vi "ex5_for loop.vi"() -> ()   [LabVIEW 2018]
panel:
  out "Numeric 2":dbl
  out "Array":dbl[](array[numeric])
  out "Numeric":dbl
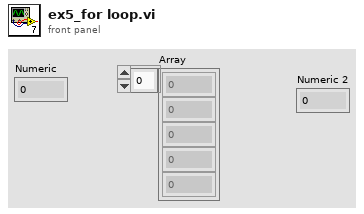
[diagram p1: front panel]
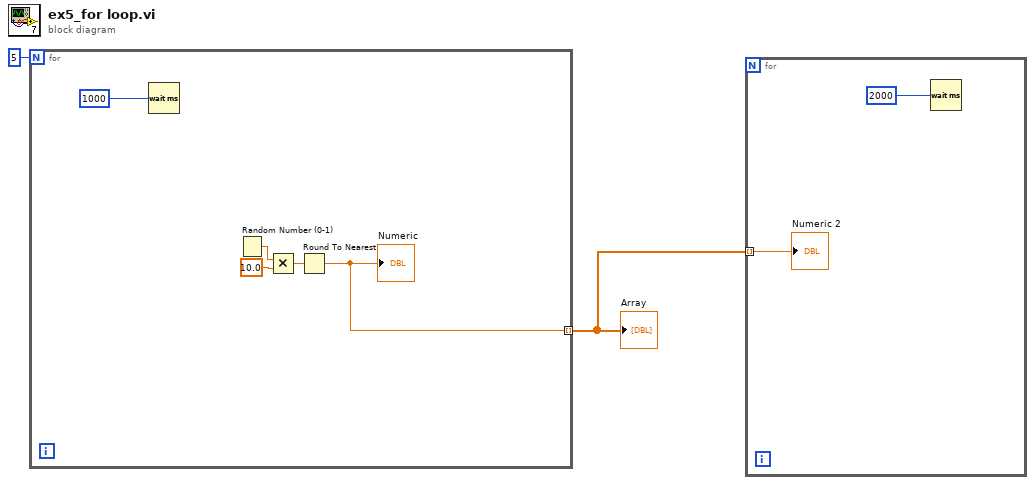
[diagram p0: block diagram]
diagram:
  n1 = for {
    N: 5 -> [_]
    tunnel: [w3] -> w1 mode=indexing
    n2 = Wait (ms)(milliseconds to wait=u32 1000 ("millisecond timer value")) -> ()  [unwired: 1 out]
    n3 = Random Number (0-1)() -> (number: 0 to 1=w6:dbl)
    n4 = Multiply(x=w6, y=10.0) -> (x*y=w7:dbl)
    n5 = Round To Nearest(number=w7) -> (nearest integer value=w3:dbl)
    "Numeric" <- w3
  }
  "Array" <- w1
  n6 = for {
    tunnel: w1 -> [w8] mode=indexing
    n7 = Wait (ms)(milliseconds to wait=u32 2000 ("millisecond timer value")) -> ()  [unwired: 1 out]
    "Numeric 2" <- w8
  }
